vi "oa_Check DC Gap Input Data (1 Channel).vi"(0 "even angle signal":cluster{"r0":dbl, "dr":dbl, "Y":dbl[]}={"r0"=0.0, "dr"=1.0, "Y"=[]} {"r0" format="%.2p"; "dr" format="%.2p"; "Y" format="%.2f"}, 1 "reset":bool=TRUE, 5 "averaging type":enum16{"Linear", "Exponential"}(ring), 7 "window":T1(ring), 9 "DC gap reference [V]":dbl=inf, 11 "error in (no error)":errorcluster) -> (2 "DC ref changed?":bool, 3 "reset?":bool, 4 "even angle signal":cluster{"r0":dbl, "dr":dbl, "Y":dbl[]}={"r0"=0.0, "dr"=1.0, "Y"=[]} {"r0" format="%.2p"; "dr" format="%.2p"; "Y" format="%.2f"}, 6 "averaging type out":enum16{"Linear", "Exponential"}(ring), 8 "window out":T1(ring), 10 "DC gap reference [V] out":dbl=inf, 15 "error out":errorcluster)   [LabVIEW 2017, in "SoundVib_RefDataProcess.lvlib"]
uses:
  <vilib>/addons/Sound and Vibration/Order Analysis/Referece Data Processing/SoundVib_RefDataProcess.lvlib
  <vilib>/addons/Sound and Vibration/Order Analysis/Resample Order Tracking/SubVIs/OAT Verify Resampled Signal (Single Channel).vi
  <vilib>/addons/Sound and Vibration/Order Analysis/Resample Order Tracking/SoundVib_Resampling.lvlib
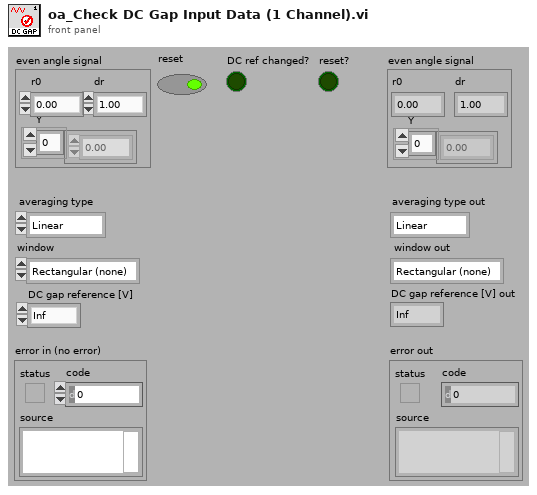
[diagram p1: front panel]
types:
  T1 = enum16{"Rectangular (none)", "Hanning", "Low side lobe"}
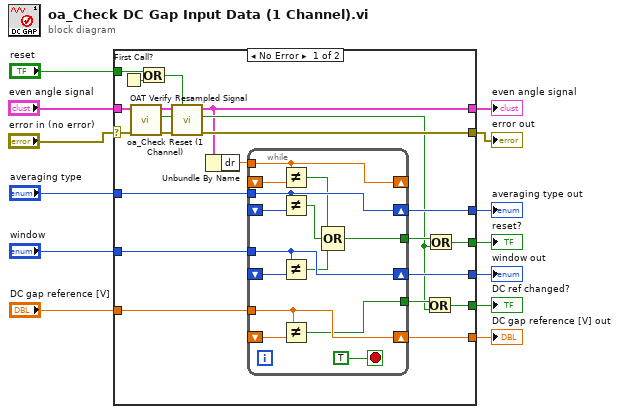
[diagram p0: block diagram]
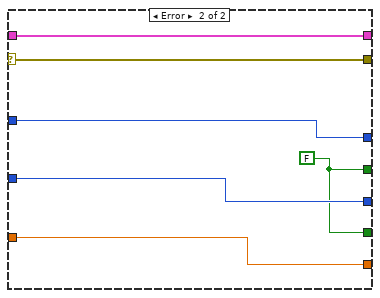
[diagram p2: hidden frame]
diagram:
  n1 = case shown="No Error" "error in (no error)" {
    selector: "error in (no error)" -> [w25 w55]
    tunnel: [w17 w55] -> w12
    tunnel: "window" -> [w35 w52]
    tunnel: "averaging type" -> [w34 w53]
    tunnel: [w33 w53] -> w9
    tunnel: [w32 w52] -> w8
    tunnel: [w22 w51] -> w7
    tunnel: "even angle signal" -> [w26 w54]
    tunnel: [w14 w54] -> w5
    tunnel: "DC gap reference [V]" -> [w30 w50]
    tunnel: [w29 w50] -> w3
    tunnel: [w21 w51] -> w2
    tunnel: "reset" -> [w24 _]
    frame No Error {
      n2 = First Call?() -> (First Call?: T/F=w23:bool)
      n3 = call-poly <vilib>:"OAT Verify Resampled Signal.vi"("error in (no error)"=w25, "resampled signal"=w26) -> ("error out"=w18:errorcluster, "empty signal?"=w20:bool, "resampled signal dup"=w19:cluster{"r0":dbl, "dr":dbl, "Y":dbl[]})  [unwired: 7 in]
      n4 = Or(x=w24, y=w23) -> (x .or. y?=w15:bool)
      n5 = call <vilib>:"oa_Check Reset (1 Channel).vi"("reset?"=w15, "error in (no error)"=w18, "empty signal?"=w20, "resampled signal"=w19) -> ("error out"=w17:errorcluster, "reset out?"=w16:bool, "resampled signal dup"=w14:cluster{"r0":dbl, "dr":dbl, "Y":dbl[]})  [unwired: 5 in]
      n6 = Unbundle By Name(w14) -> ("dr"=w27:dbl)
      n7 = while {
        tunnel: w35 -> [w46]
        tunnel: w34 -> [w48]
        shift-right: [w48] -> w33
        shift-left: _ -> [w47]
        shift-right: [w46] -> w32
        shift-left: _ -> [w45]
        tunnel: [w39] -> w31
        tunnel: w27 -> [w44]
        shift-right: [w44] -> _
        shift-left: _ -> [w43]
        tunnel: w30 -> [w38]
        shift-right: [w38] -> w29
        shift-left: _ -> [w37]
        tunnel: [w36] -> w28
        stop <- TRUE stop-if-true
        n8 = Not Equal?(x=w44, y=w43) -> (x != y?=w42:bool)
        n9 = Not Equal?(x=w48, y=w47) -> (x != y?=w41:bool)
        n10 = Not Equal?(x=w46, y=w45) -> (x != y?=w40:bool)
        n11 = Not Equal?(x=w38, y=w37) -> (x != y?=w36:bool)
        n12 = Compound Arithmetic op=OR(w42, w41, w40) -> (w39:bool)
      }
      n13 = Or(x=w28, y=w16) -> (x .or. y?=w21:bool)
      n14 = Or(x=w31, y=w16) -> (x .or. y?=w22:bool)
    }
    frame Error {
      w51 = FALSE
    }
  }
  "error out" <- w12
  "even angle signal" <- w5
  "averaging type out" <- w9
  "window out" <- w8
  "reset?" <- w7
  "DC gap reference [V] out" <- w3
  "DC ref changed?" <- w2
